vi "Run.vi"(8 "error in (no error)":errorcluster, 11 "Channel in":refnum<class "Channel.lvclass">) -> (0 "error out":errorcluster, 3 "Channel out":refnum<class "Channel.lvclass">)   [LabVIEW 2018, in "Channel.lvclass"]
doc: "Run the channel"
uses:
  Channel.lvclass
  Channel.lvclass/Channel.ctl
  Header content/Header content.lvclass/Header content.ctl
  Server/Server.lvclass/Server.ctl
  Simulated_CCD_Camera/Simulated Camera.lvclass/Simulated Camera.ctl
  Server/Server.lvclass
  RxTx/CCS_RxTx.lvclass
  State Machine/CCS_State Machine.lvclass
  Simulated_CCD_Camera/Simulated Camera.lvclass
  Header content/Header content.lvclass
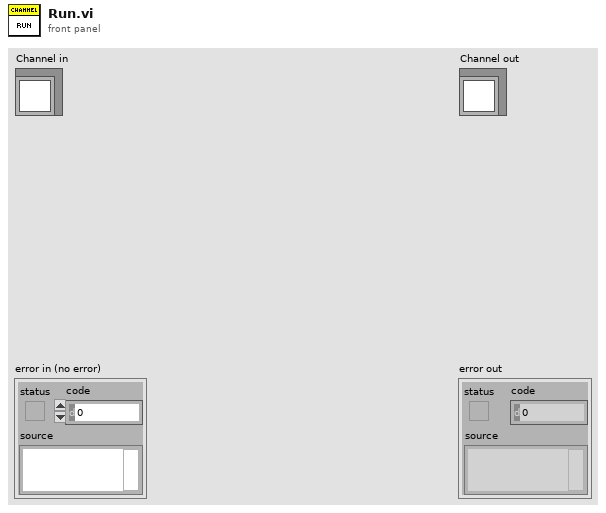
[diagram p1: front panel]
types:
  T1 = cluster{"PREAMP":u16, "READOUT_RATE":u16, "EM_GAIN":u16, "VERTICAL_SHIFT_SPEED":u16, "READ_MODE":u16, "FRAME_TRANSFER":bool, "VERTICAL_CLOCK_VOLTAGE":u16, "ACQUISITION_MODE":u16, "AD_CHANNEL":u16, "EM_MODE":u16, "SHUTTER_TTL":u16, "SHUTTER_OPENING_TIME":u16, "SHUTTER_CLOSING_TIME":u16, "SHUTTER_MODE":u16, "TRIGGER_MODE":u16, "VBIN":u16, "INITIAL_LINE":u16, "INITIAL_COLUMN":u16, "FINAL_LINE":u16, "FINAL_COLUMN":u16, "HBIN":u16}
  T2 = cluster{"CYCLES_DONE":u16, "LAST_IMAGE_NAME":string, "USED_DISK_SPACE":u16, "FRAMES_DONE":u16, "CCD_STATUS":string, "CURRENT_TEMPERATURE":i16, "TEMPERATURE_STATUS":string, "FRAME_EXPOSURE_TIME":sgl, "ERROR":bool, "SERIAL_NUMBER":u16, "ACQUIRING":bool, "IMAGE_INDEX":u32, "SEQS_DONE":u16}
  T3 = cluster{"COOLER_POWER_STATUS":u16, "TEMP":i32, "EXPTIME":dbl, "#FRAMES":u32, "#CYCLES":u32, "#SEQS":u32, "WAVEPLATE_POS":u16}
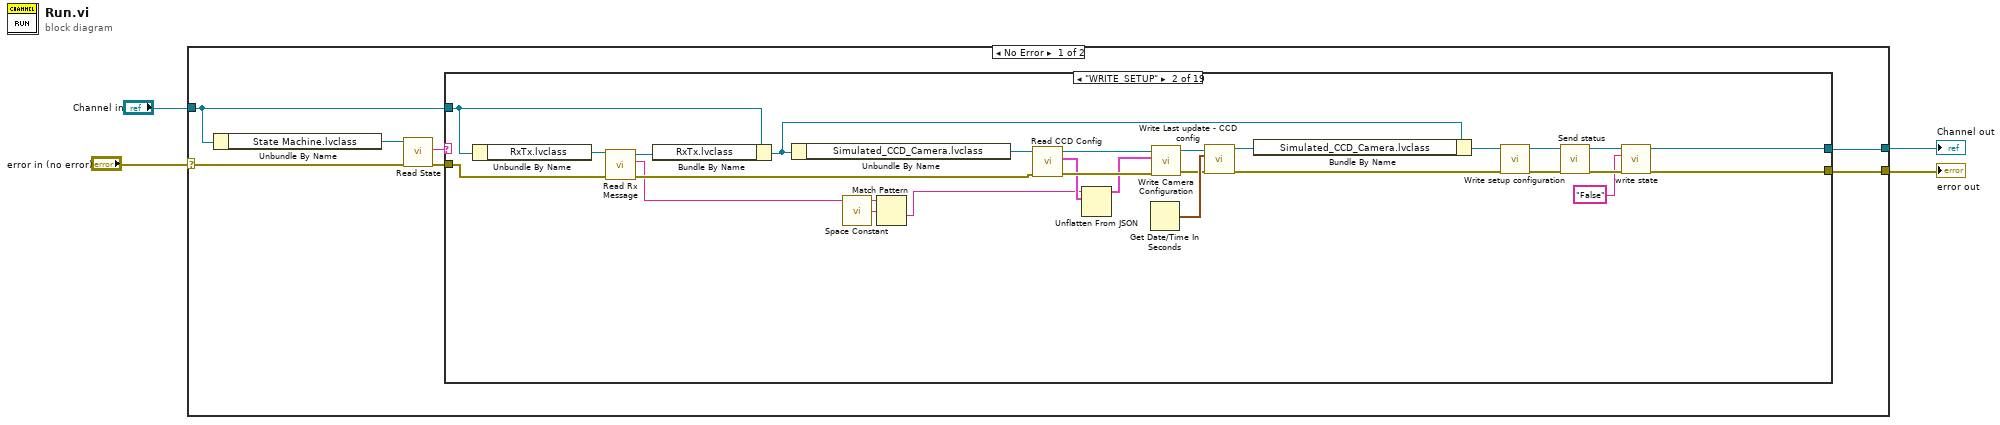
[diagram p0: block diagram]
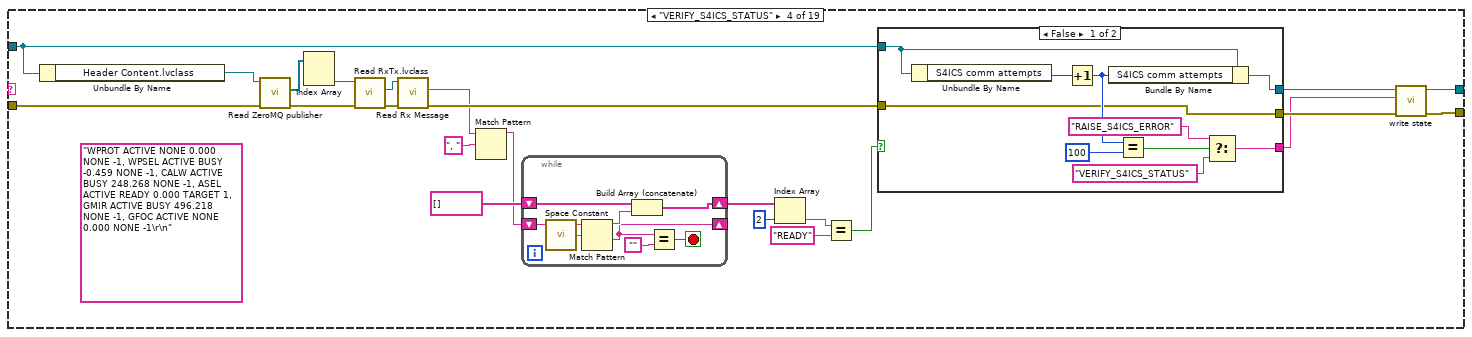
[diagram p4: hidden frame]
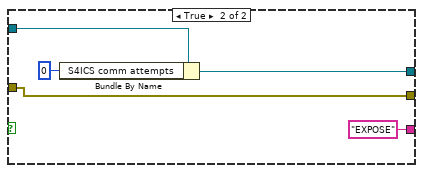
[diagram p5: hidden frame]
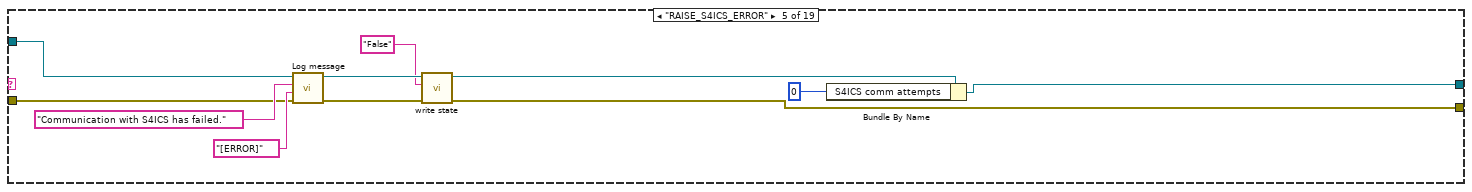
[diagram p6: hidden frame]
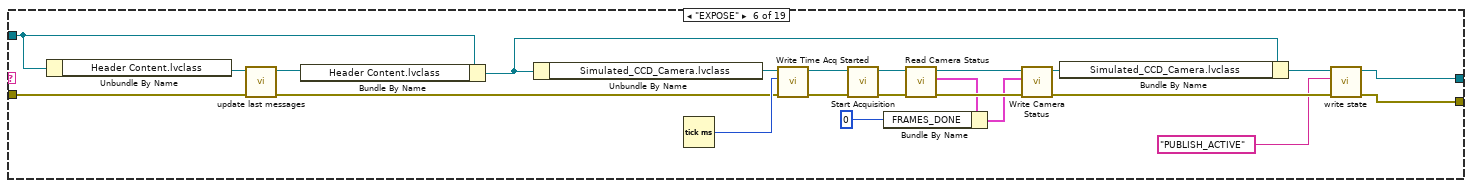
[diagram p7: hidden frame]
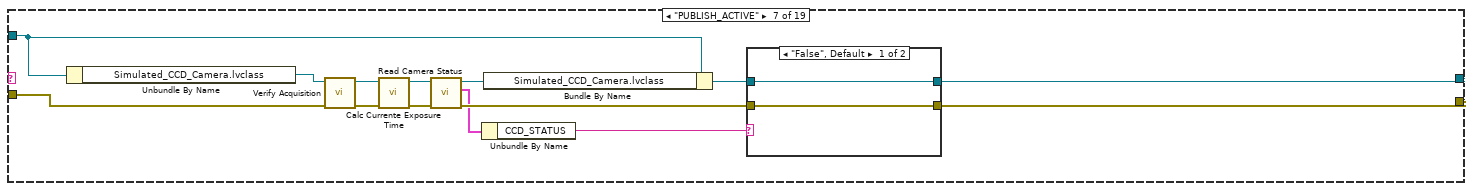
[diagram p8: hidden frame]
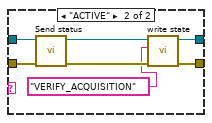
[diagram p9: hidden frame]
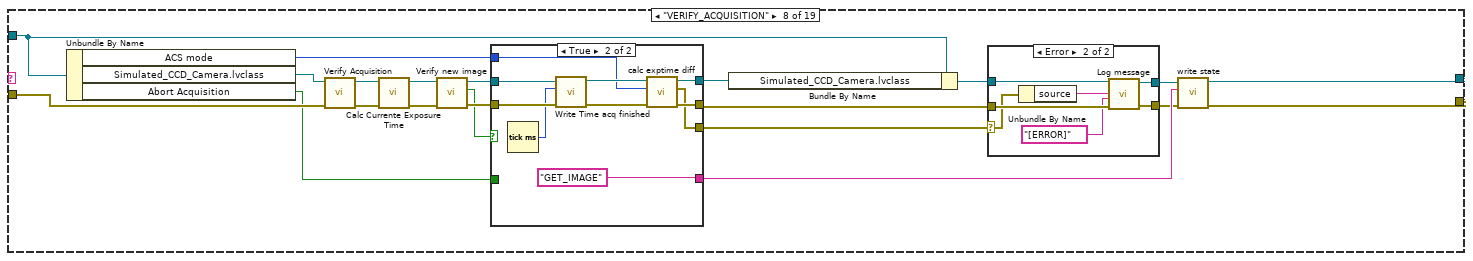
[diagram p10: hidden frame]
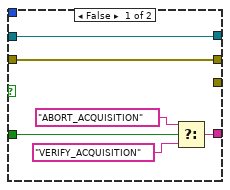
[diagram p12: hidden frame]
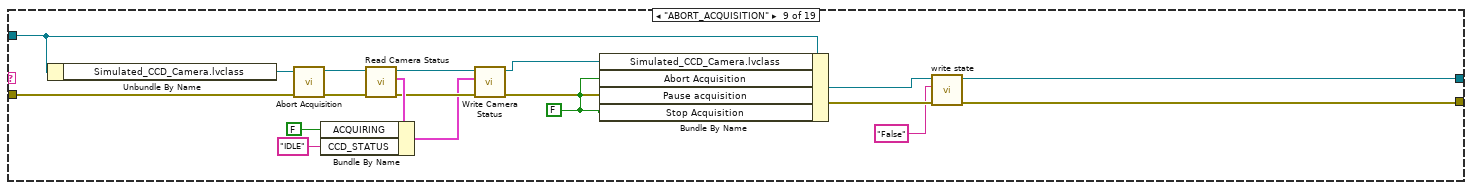
[diagram p13: hidden frame]
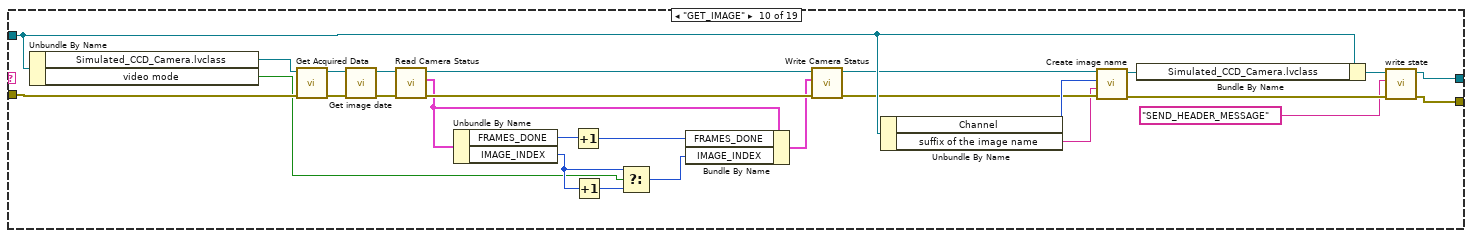
[diagram p14: hidden frame]
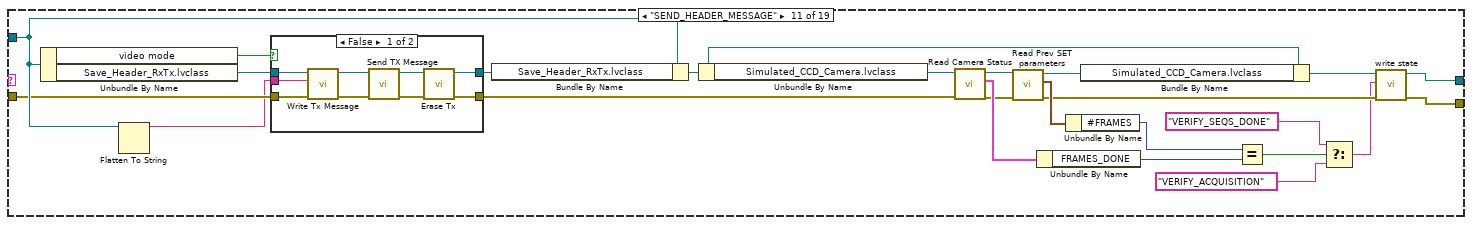
[diagram p15: hidden frame]
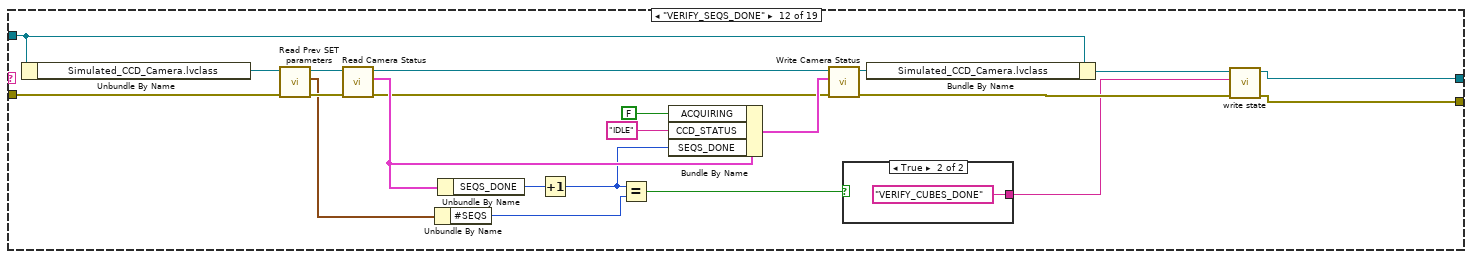
[diagram p17: hidden frame]
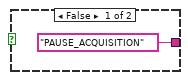
[diagram p18: hidden frame]
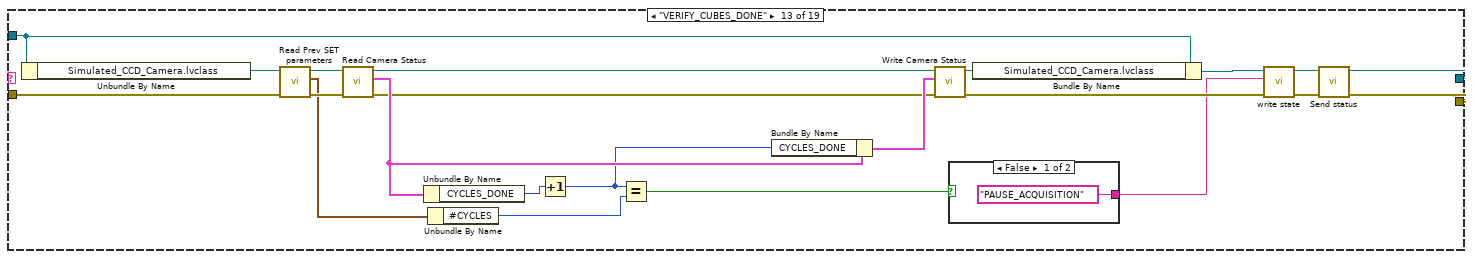
[diagram p19: hidden frame]
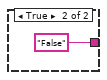
[diagram p20: hidden frame]
diagram:
  n1 = case shown="No Error" "error in (no error)" {
    selector: "error in (no error)" -> [w7 w489]
    tunnel: [w11 w489] -> w3
    tunnel: [w9 w488] -> w1
    tunnel: "Channel in" -> [w10 w488]
    frame No Error {
      n2 = Unbundle By Name(w10) -> ("State Machine.lvclass"=w8:refnum<class "CCS_State Machine.lvclass">)
      n3 = call-dynamic "Read State.vi"("error in (no error)"=w7, "State Machine in"=w8) -> ("error out"=w6:errorcluster, "State"=w5:string)  [unwired: 7 in, 1 out]
      n4 = case shown="\"WRITE_SETUP\"" w5 {
        tunnel: w6 -> [w12 w38 w41 w60 w96 w113 w133 w162 w200 w236 w246 w284 w309 w323 w329 w353 w365 w384 w401]
        tunnel: [w12 w23 w41 w46 w90 w104 w129 w158 w193 w210 w237 w272 w301 w322 w336 w352 w366 w384 w391] -> w11
        tunnel: [w13 w24 w42 w47 w91 w105 w130 w159 w194 w211 w238 w273 w302 w321 w337 w351 w367 w385 w392] -> w9
        tunnel: w10 -> [w13 w40 w42 w50 w97 w112 w136 w166 w199 w229 w248 w288 w315 w324 w349 w354 w364 w385 w403]
        frame "False", Default {
        }
        frame "WRITE_SETUP" {
          n5 = Unbundle By Name(w40) -> ("RxTx.lvclass"=w39:refnum<class "CCS_RxTx.lvclass">)
          n6 = call "Read Rx Message.vi"("error in (no error)"=w38, "RxTx in"=w39) -> ("error out"=w33:errorcluster, "Rx Message"=w15:string, "RxTx out"=w37:refnum<class "CCS_RxTx.lvclass">)  [unwired: 7 in]
          n7 = Bundle By Name(cluster=w40, "RxTx.lvclass"=w37) -> (w28:refnum<class "Channel.lvclass">)
          n8 = Unbundle By Name(w28) -> ("Simulated_CCD_Camera.lvclass"=w36:refnum<class "Simulated Camera.lvclass">)
          n9 = call <vilib>:"Space Constant.vi"() -> ("String"=w16:string)
          n10 = Match Pattern(string=w15, regular expression=w16) -> (after substring=w14:string)  [unwired: 1 in, 3 out]
          n11 = call "Read CCD Config.vi"("error in (no error)"=w33, "CCDCamera in"=w36) -> ("error out"=w34:errorcluster, "CCD Config"=w32:T1, "CCDCamera out"=w35:refnum<class "Simulated Camera.lvclass">)  [unwired: 7 in]
          n12 = Unflatten From JSON(JSON string=w14, type and defaults=w32) -> (value=w31:T1)  [unwired: 5 in, 1 out]
          n13 = Get Date/Time In Seconds() -> (seconds since 1Jan1904=w30:timestamp)
          n14 = call-dynamic "Write Camera Configuration.vi"("error in (no error)"=w34, "CCD Config"=w31, "CCDCamera in"=w35) -> ("error out"=w21:errorcluster, "CCDCamera out"=w22:refnum<class "Simulated Camera.lvclass">)  [unwired: 7 in]
          n15 = call-dynamic "Write Last update - CCD config.vi"("error in (no error)"=w21, "Last update - CCD config"=w30, "Simulated_CCD_Camera in"=w22) -> ("error out"=w19:errorcluster, "Simulated_CCD_Camera out"=w29:refnum<class "Simulated Camera.lvclass">)  [unwired: 7 in]
          n16 = Bundle By Name(cluster=w28, "Simulated_CCD_Camera.lvclass"=w29) -> (w20:refnum<class "Channel.lvclass">)
          n17 = call "Write setup configuration.vi"("error in (no error)"=w19, "Channel in"=w20) -> ("error out"=w18:errorcluster, "Channel out"=w17:refnum<class "Channel.lvclass">)  [unwired: 8 in]
          n18 = call "Send status.vi"("error in (no error)"=w18, "Channel in"=w17) -> ("error out"=w26:errorcluster, "Channel out"=w27:refnum<class "Channel.lvclass">)  [unwired: 8 in]
          n19 = call "write state.vi"("error in (no error)"=w26, "state"="False", "Channel in"=w27) -> ("error out"=w23:errorcluster, "Channel out"=w24:refnum<class "Channel.lvclass">)  [unwired: 7 in]
        }
        frame "---------------------------------" {
        }
        frame "VERIFY_S4ICS_STATUS" {
          (unwired) "WPROT ACTIVE NONE 0.000 NONE -1, WPSEL ACTIVE BUSY -0.459 NONE -1, CALW ACTIVE BUSY 248.268 NONE -1, ASEL ACTIVE READY 0.000 TARGET 1, GMIR ACTIVE BUSY 496.218 NONE -1, GFOC ACTIVE NONE 0.000 NONE -1\r\n" ("search string/char (-)")
          n20 = Unbundle By Name(w50) -> ("Header Content.lvclass"=w59:refnum<class "Header content.lvclass">)
          n21 = call "Read ZeroMQ publisher.vi"("error in (no error)"=w60, "Header content in"=w59) -> ("error out"=w62:errorcluster, "ZeroMQ publisher"=w65:refnum<class "Server.lvclass">[])  [unwired: 7 in, 1 out]
          n22 = Index Array(array=w65) -> (element #2=w61:refnum<class "Server.lvclass">)  [unwired: 2 in, 1 out]
          n23 = call "Read RxTx.lvclass.vi"("error in (no error)"=w62, "Server in"=w61) -> ("error out"=w63:errorcluster, "RxTx.lvclass"=w64:refnum<class "CCS_RxTx.lvclass">)  [unwired: 7 in, 1 out]
          n24 = call "Read Rx Message.vi"("error in (no error)"=w63, "RxTx in"=w64) -> ("error out"=w49:errorcluster, "Rx Message"=w43:string)  [unwired: 7 in, 1 out]
          n25 = Match Pattern(string=w43, regular expression=", " ("search string/char (-)")) -> (before substring=w56:string)  [unwired: 1 in, 3 out]
          n26 = while {
            shift-right: [w85] -> w52
            shift-left: string[] [] -> [w86]
            shift-right: [w82] -> _
            shift-left: w56 -> [w84]
            stop <- w87 stop-if-true
            n27 = call <vilib>:"Space Constant.vi"() -> ("String"=w81:string)
            n28 = Match Pattern(string=w84, regular expression=w81) -> (before substring=w83:string, after substring=w82:string)  [unwired: 1 in, 2 out]
            n29 = Build Array (concatenate)(w86, w83) -> (w85:string[])
            n30 = Equal?(x=w82, y="") -> (x = y?=w87:bool)
          }
          n31 = Index Array(array=w52, index=2) -> (element=w54:string)
          n32 = Equal?(x=w54, y="READY") -> (x = y?=w51:bool)
          n33 = case shown="False" w51 {
            tunnel: w50 -> [w75 w80]
            tunnel: w49 -> [w68 w79]
            tunnel: [w67 w78] -> w48
            tunnel: [w68 w79] -> w45
            tunnel: [w66 "EXPOSE" ("y")] -> w44
            frame False {
              n34 = Unbundle By Name(w75) -> ("S4ICS comm attempts"=w74:u8)
              n35 = Increment(x=w74) -> (x+1=w73:u8)
              n36 = Bundle By Name(cluster=w75, "S4ICS comm attempts"=w73) -> (w67:refnum<class "Channel.lvclass">)
              n37 = Equal?(x=w73, y=100) -> (x = y?=w71:bool)
              n38 = Select(t="RAISE_S4ICS_ERROR" ("y"), s=w71, f="VERIFY_S4ICS_STATUS" ("y")) -> (s? t:f=w66:string)
            }
            frame True {
              n39 = Bundle By Name(cluster=w80, "S4ICS comm attempts"=u8 0) -> (w78:refnum<class "Channel.lvclass">)
            }
          }
          n40 = call "write state.vi"("error in (no error)"=w45, "state"=w44, "Channel in"=w48) -> ("error out"=w46:errorcluster, "Channel out"=w47:refnum<class "Channel.lvclass">)  [unwired: 7 in]
        }
        frame "RAISE_S4ICS_ERROR" {
          n41 = call "Log message.vi"("error in (no error)"=w96, "message type"="[ERROR]", "String"="Communication with S4ICS has failed.", "Channel in"=w97) -> ("error out"=w93:errorcluster, "Channel out"=w94:refnum<class "Channel.lvclass">)  [unwired: 6 in]
          n42 = call "write state.vi"("error in (no error)"=w93, "state"="False", "Channel in"=w94) -> ("error out"=w90:errorcluster, "Channel out"=w92:refnum<class "Channel.lvclass">)  [unwired: 7 in]
          n43 = Bundle By Name(cluster=w92, "S4ICS comm attempts"=u8 0) -> (w91:refnum<class "Channel.lvclass">)
        }
        frame "EXPOSE" {
          n44 = Unbundle By Name(w112) -> ("Header Content.lvclass"=w114:refnum<class "Header content.lvclass">)
          n45 = call "update last messages.vi"("error in (no error)"=w113, "Header content in"=w114) -> ("error out"=w110:errorcluster, "Header content out"=w111:refnum<class "Header content.lvclass">)  [unwired: 8 in]
          n46 = Bundle By Name(cluster=w112, "Header Content.lvclass"=w111) -> (w109:refnum<class "Channel.lvclass">)
          n47 = Unbundle By Name(w109) -> ("Simulated_CCD_Camera.lvclass"=w122:refnum<class "Simulated Camera.lvclass">)
          n48 = Tick Count (ms)() -> (millisecond timer value=w121:u32)
          n49 = call "Write Time Acq Started.vi"("error in (no error)"=w110, "Time Acq Started"=w121, "Simulated_CCD_Camera in"=w122) -> ("error out"=w100:errorcluster, "Simulated_CCD_Camera out"=w103:refnum<class "Simulated Camera.lvclass">)  [unwired: 7 in]
          n50 = call-dynamic "Start Acquisition.vi"("error in (no error)"=w100, "CCDCamera in"=w103) -> ("error out"=w101:errorcluster, "CCDCamera out"=w102:refnum<class "Simulated Camera.lvclass">)  [unwired: 8 in]
          n51 = call "Read Camera Status.vi"("error in (no error)"=w101, "CCDCamera in"=w102) -> ("error out"=w119:errorcluster, "Camera Status"=w117:T2, "CCDCamera out"=w118:refnum<class "Simulated Camera.lvclass">)  [unwired: 7 in]
          n52 = Bundle By Name(cluster=w117, "FRAMES_DONE"=u16 0) -> (w116:T2)
          n53 = call "Write Camera Status.vi"("error in (no error)"=w119, "Camera Status"=w116, "CCDCamera in"=w118) -> ("error out"=w107:errorcluster, "CCDCamera out"=w120:refnum<class "Simulated Camera.lvclass">)  [unwired: 7 in]
          n54 = Bundle By Name(cluster=w109, "Simulated_CCD_Camera.lvclass"=w120) -> (w108:refnum<class "Channel.lvclass">)
          n55 = call "write state.vi"("error in (no error)"=w107, "state"="PUBLISH_ACTIVE", "Channel in"=w108) -> ("error out"=w104:errorcluster, "Channel out"=w105:refnum<class "Channel.lvclass">)  [unwired: 7 in]
        }
        frame "PUBLISH_ACTIVE" {
          n56 = Unbundle By Name(w136) -> ("Simulated_CCD_Camera.lvclass"=w134:refnum<class "Simulated Camera.lvclass">)
          n57 = call-dynamic "Verify Acquisition.vi"("error in (no error)"=w133, "CCDCamera in"=w134) -> ("error out"=w135:errorcluster, "CCDCamera out"=w132:refnum<class "Simulated Camera.lvclass">)  [unwired: 8 in]
          n58 = call-dynamic "Calc Currente Exposure Time.vi"("error in (no error)"=w135, "CCDCamera in"=w132) -> ("error out"=w128:errorcluster, "CCDCamera out"=w127:refnum<class "Simulated Camera.lvclass">)  [unwired: 8 in]
          n59 = call "Read Camera Status.vi"("error in (no error)"=w128, "CCDCamera in"=w127) -> ("error out"=w125:errorcluster, "Camera Status"=w124:T2, "CCDCamera out"=w126:refnum<class "Simulated Camera.lvclass">)  [unwired: 7 in]
          n60 = Unbundle By Name(w124) -> ("CCD_STATUS"=w123:string)
          n61 = Bundle By Name(cluster=w136, "Simulated_CCD_Camera.lvclass"=w126) -> (w131:refnum<class "Channel.lvclass">)
          n62 = case shown="\"False\", Default" w123 {
            tunnel: w131 -> [w138 w141]
            tunnel: [w138 w145] -> w130
            tunnel: [w137 w144] -> w129
            tunnel: w125 -> [w137 w140]
            frame "False", Default {
            }
            frame "ACTIVE" {
              n63 = call "Send status.vi"("error in (no error)"=w140, "Channel in"=w141) -> ("error out"=w143:errorcluster, "Channel out"=w142:refnum<class "Channel.lvclass">)  [unwired: 8 in]
              n64 = call "write state.vi"("error in (no error)"=w143, "state"="VERIFY_ACQUISITION", "Channel in"=w142) -> ("error out"=w144:errorcluster, "Channel out"=w145:refnum<class "Channel.lvclass">)  [unwired: 7 in]
            }
          }
        }
        frame "VERIFY_ACQUISITION" {
          n65 = Unbundle By Name(w166) -> ("ACS mode"=w151:u16, "Simulated_CCD_Camera.lvclass"=w163:refnum<class "Simulated Camera.lvclass">, "Abort Acquisition"=w154:bool)
          n66 = call-dynamic "Verify Acquisition.vi"("error in (no error)"=w162, "CCDCamera in"=w163) -> ("error out"=w164:errorcluster, "CCDCamera out"=w161:refnum<class "Simulated Camera.lvclass">)  [unwired: 8 in]
          n67 = call-dynamic "Calc Currente Exposure Time.vi"("error in (no error)"=w164, "CCDCamera in"=w161) -> ("error out"=w165:errorcluster, "CCDCamera out"=w160:refnum<class "Simulated Camera.lvclass">)  [unwired: 8 in]
          n68 = call-dynamic "Verify new image.vi"("error in (no error)"=w165, "CCDCamera in"=w160) -> ("error out"=w156:errorcluster, "New Images ?"=w153:bool, "CCDCamera out"=w157:refnum<class "Simulated Camera.lvclass">)  [unwired: 7 in]
          n69 = case shown="True" w153 {
            tunnel: w157 -> [w181 w191]
            tunnel: w156 -> [w180 w190]
            tunnel: [w181 w185] -> w155
            tunnel: [w180 w186] -> w147
            tunnel: w154 -> [w177 _]
            tunnel: [w176 "GET_IMAGE"] -> w152
            tunnel: w151 -> [_ w183]
            tunnel: [_ w182] -> w146
            frame False {
              n70 = Select(t="ABORT_ACQUISITION", s=w177, f="VERIFY_ACQUISITION") -> (s? t:f=w176:string)
            }
            frame True {
              n71 = Tick Count (ms)() -> (millisecond timer value=w188:u32)
              n72 = call "Write Time acq finished.vi"("error in (no error)"=w190, "Time acq finished"=w188, "Simulated_CCD_Camera in"=w191) -> ("error out"=w187:errorcluster, "Simulated_CCD_Camera out"=w184:refnum<class "Simulated Camera.lvclass">)  [unwired: 7 in]
              n73 = call "calc exptime diff.vi"("error in (no error)"=w187, "ACS mode"=w183, "Simulated_CCD_Camera in"=w184) -> (0:"error out"=w186:errorcluster, 2:"error out"=w182:errorcluster, "Simulated_CCD_Camera out"=w185:refnum<class "Simulated Camera.lvclass">)  [unwired: 6 in]
            }
          }
          n74 = Bundle By Name(cluster=w166, "Simulated_CCD_Camera.lvclass"=w155) -> (w150:refnum<class "Channel.lvclass">)
          n75 = case shown="Error" w146 {
            selector: w146 -> [_ w170]
            tunnel: w150 -> [w168 w175]
            tunnel: [w168 w174] -> w149
            tunnel: [w167 w173] -> w148
            tunnel: w147 -> [w167 w172]
            frame No Error {
            }
            frame Error {
              n76 = Unbundle By Name(w170) -> ("source"=w169:string)
              n77 = call "Log message.vi"("error in (no error)"=w172, "message type"="[ERROR]", "String"=w169, "Channel in"=w175) -> ("error out"=w173:errorcluster, "Channel out"=w174:refnum<class "Channel.lvclass">)  [unwired: 6 in]
            }
          }
          n78 = call "write state.vi"("error in (no error)"=w148, "state"=w152, "Channel in"=w149) -> ("error out"=w158:errorcluster, "Channel out"=w159:refnum<class "Channel.lvclass">)  [unwired: 7 in]
        }
        frame "ABORT_ACQUISITION" {
          w192 = FALSE ("Acquiring")
          n79 = Unbundle By Name(w199) -> ("Simulated_CCD_Camera.lvclass"=w201:refnum<class "Simulated Camera.lvclass">)
          n80 = call-dynamic "Abort Acquisition.vi"("error in (no error)"=w200, "CCDCamera in"=w201) -> ("error out"=w206:errorcluster, "CCDCamera out"=w207:refnum<class "Simulated Camera.lvclass">)  [unwired: 8 in]
          n81 = call "Read Camera Status.vi"("error in (no error)"=w206, "CCDCamera in"=w207) -> ("error out"=w204:errorcluster, "Camera Status"=w209:T2, "CCDCamera out"=w205:refnum<class "Simulated Camera.lvclass">)  [unwired: 7 in]
          n82 = Bundle By Name(cluster=w209, "ACQUIRING"=FALSE ("Acquiring"), "CCD_STATUS"="IDLE" ("STATUS")) -> (w203:T2)
          n83 = call "Write Camera Status.vi"("error in (no error)"=w204, "Camera Status"=w203, "CCDCamera in"=w205) -> ("error out"=w196:errorcluster, "CCDCamera out"=w198:refnum<class "Simulated Camera.lvclass">)  [unwired: 7 in]
          n84 = Bundle By Name(cluster=w199, "Simulated_CCD_Camera.lvclass"=w198, "Abort Acquisition"=w192, "Pause acquisition"=w192, "Stop Acquisition"=w192) -> (w197:refnum<class "Channel.lvclass">)
          n85 = call "write state.vi"("error in (no error)"=w196, "state"="False", "Channel in"=w197) -> ("error out"=w193:errorcluster, "Channel out"=w194:refnum<class "Channel.lvclass">)  [unwired: 7 in]
        }
        frame "GET_IMAGE" {
          n86 = Unbundle By Name(w229) -> ("Simulated_CCD_Camera.lvclass"=w218:refnum<class "Simulated Camera.lvclass">, "video mode"=w215:bool)
          n87 = call-dynamic "Get Acquired Data.vi"("error in (no error)"=w236, "CCDCamera in"=w218) -> ("error out"=w221:errorcluster, "CCDCamera out"=w224:refnum<class "Simulated Camera.lvclass">)  [unwired: 8 in]
          n88 = call-dynamic "Get image date.vi"("error in (no error)"=w221, "Simulated_CCD_Camera in"=w224) -> ("error out"=w222:errorcluster, "Simulated_CCD_Camera out"=w223:refnum<class "Simulated Camera.lvclass">)  [unwired: 8 in]
          n89 = call "Read Camera Status.vi"("error in (no error)"=w222, "CCDCamera in"=w223) -> ("error out"=w235:errorcluster, "Camera Status"=w231:T2, "CCDCamera out"=w234:refnum<class "Simulated Camera.lvclass">)  [unwired: 7 in]
          n90 = Unbundle By Name(w231) -> ("FRAMES_DONE"=w233:u16, "IMAGE_INDEX"=w216:u32)
          n91 = Increment(x=w233) -> (x+1=w219:u16)
          n92 = Increment(x=w216) -> (x+1=w217:u32)
          n93 = Select(t=w216, s=w215, f=w217) -> (s? t:f=w220:u32)
          n94 = Bundle By Name(cluster=w231, "FRAMES_DONE"=w219, "IMAGE_INDEX"=w220) -> (w232:T2)
          n95 = call "Write Camera Status.vi"("error in (no error)"=w235, "Camera Status"=w232, "CCDCamera in"=w234) -> ("error out"=w226:errorcluster, "CCDCamera out"=w227:refnum<class "Simulated Camera.lvclass">)  [unwired: 7 in]
          n96 = Unbundle By Name(w229) -> ("Channel"=w228:u8, "suffix of the image name"=w225:string)
          n97 = call "Create image name.vi"("error in (no error)"=w226, "Suffix"=w225, "Channel"=w228, "Simulated_CCD_Camera in"=w227) -> ("error out"=w213:errorcluster, "Simulated_CCD_Camera out"=w230:refnum<class "Simulated Camera.lvclass">)  [unwired: 6 in]
          n98 = Bundle By Name(cluster=w229, "Simulated_CCD_Camera.lvclass"=w230) -> (w214:refnum<class "Channel.lvclass">)
          n99 = call "write state.vi"("error in (no error)"=w213, "state"="SEND_HEADER_MESSAGE", "Channel in"=w214) -> ("error out"=w210:errorcluster, "Channel out"=w211:refnum<class "Channel.lvclass">)  [unwired: 7 in]
        }
        frame "SEND_HEADER_MESSAGE" {
          n100 = Unbundle By Name(w248) -> ("video mode"=w242:bool, "Save_Header_RxTx.lvclass"=w247:refnum<class "CCS_RxTx.lvclass">)
          n101 = Flatten To String(anything=w248) -> (data string=w243:string)  [unwired: 3 in, 2 out]
          n102 = case shown="False" w242 {
            tunnel: w247 -> [w269 w271]
            tunnel: w246 -> [w266 w270]
            tunnel: [w264 w271] -> w245
            tunnel: [w262 w270] -> w244
            tunnel: w243 -> [w261 _]
            frame False {
              n103 = call "Write Tx Message.vi"("error in (no error)"=w266, "Tx Message"=w261, "RxTx in"=w269) -> ("error out"=w267:errorcluster, "RxTx out"=w268:refnum<class "CCS_RxTx.lvclass">)  [unwired: 7 in]
              n104 = call "Send TX Message.vi"("error in (no error)"=w267, "RxTx in"=w268) -> ("error out"=w263:errorcluster, "RxTx out"=w265:refnum<class "CCS_RxTx.lvclass">)  [unwired: 8 in]
              n105 = call "Erase Tx.vi"("error in (no error)"=w263, "RxTx in"=w265) -> ("error out"=w262:errorcluster, "RxTx out"=w264:refnum<class "CCS_RxTx.lvclass">)  [unwired: 8 in]
            }
            frame True {
            }
          }
          n106 = Bundle By Name(cluster=w248, "Save_Header_RxTx.lvclass"=w245) -> (w258:refnum<class "Channel.lvclass">)
          n107 = Unbundle By Name(w258) -> ("Simulated_CCD_Camera.lvclass"=w255:refnum<class "Simulated Camera.lvclass">)
          n108 = call "Read Camera Status.vi"("error in (no error)"=w244, "CCDCamera in"=w255) -> ("error out"=w251:errorcluster, "Camera Status"=w254:T2, "CCDCamera out"=w253:refnum<class "Simulated Camera.lvclass">)  [unwired: 7 in]
          n109 = call-dynamic "Read Prev SET parameters.vi"("error in (no error)"=w251, "Simulated_CCD_Camera in"=w253) -> ("error out"=w240:errorcluster, "Prev SET parameters"=w250:T3, "Simulated_CCD_Camera out"=w252:refnum<class "Simulated Camera.lvclass">)  [unwired: 7 in]
          n110 = Unbundle By Name(w254) -> ("FRAMES_DONE"=w260:u16)
          n111 = Unbundle By Name(w250) -> ("#FRAMES"=w249:u32)
          n112 = Bundle By Name(cluster=w258, "Simulated_CCD_Camera.lvclass"=w252) -> (w241:refnum<class "Channel.lvclass">)
          n113 = Equal?(x=w249, y=w260) -> (x = y?=w259:bool)
          n114 = Select(t="VERIFY_SEQS_DONE", s=w259, f="VERIFY_ACQUISITION") -> (s? t:f=w239:string)
          n115 = call "write state.vi"("error in (no error)"=w240, "state"=w239, "Channel in"=w241) -> ("error out"=w237:errorcluster, "Channel out"=w238:refnum<class "Channel.lvclass">)  [unwired: 7 in]
        }
        frame "VERIFY_SEQS_DONE" {
          n116 = Unbundle By Name(w288) -> ("Simulated_CCD_Camera.lvclass"=w287:refnum<class "Simulated Camera.lvclass">)
          n117 = call-dynamic "Read Prev SET parameters.vi"("error in (no error)"=w284, "Simulated_CCD_Camera in"=w287) -> ("error out"=w285:errorcluster, "Prev SET parameters"=w283:T3, "Simulated_CCD_Camera out"=w286:refnum<class "Simulated Camera.lvclass">)  [unwired: 7 in]
          n118 = call "Read Camera Status.vi"("error in (no error)"=w285, "CCDCamera in"=w286) -> ("error out"=w279:errorcluster, "Camera Status"=w293:T2, "CCDCamera out"=w280:refnum<class "Simulated Camera.lvclass">)  [unwired: 7 in]
          n119 = Unbundle By Name(w283) -> ("#SEQS"=w282:u32)
          n120 = Unbundle By Name(w293) -> ("SEQS_DONE"=w292:u16)
          n121 = Increment(x=w292) -> (x+1=w290:u16)
          n122 = Equal?(x=w290, y=w282) -> (x = y?=w289:bool)
          n123 = Bundle By Name(cluster=w293, "ACQUIRING"=FALSE, "CCD_STATUS"="IDLE", "SEQS_DONE"=w290) -> (w291:T2)
          n124 = call "Write Camera Status.vi"("error in (no error)"=w279, "Camera Status"=w291, "CCDCamera in"=w280) -> ("error out"=w275:errorcluster, "CCDCamera out"=w281:refnum<class "Simulated Camera.lvclass">)  [unwired: 7 in]
          n125 = case shown="True" w289 {
            tunnel: ["PAUSE_ACQUISITION" "VERIFY_CUBES_DONE"] -> w274
            frame False {
            }
            frame True {
            }
          }
          n126 = Bundle By Name(cluster=w288, "Simulated_CCD_Camera.lvclass"=w281) -> (w276:refnum<class "Channel.lvclass">)
          n127 = call "write state.vi"("error in (no error)"=w275, "state"=w274, "Channel in"=w276) -> ("error out"=w272:errorcluster, "Channel out"=w273:refnum<class "Channel.lvclass">)  [unwired: 7 in]
        }
        frame "VERIFY_CUBES_DONE" {
          n128 = Unbundle By Name(w315) -> ("Simulated_CCD_Camera.lvclass"=w312:refnum<class "Simulated Camera.lvclass">)
          n129 = call-dynamic "Read Prev SET parameters.vi"("error in (no error)"=w309, "Simulated_CCD_Camera in"=w312) -> ("error out"=w310:errorcluster, "Prev SET parameters"=w308:T3, "Simulated_CCD_Camera out"=w311:refnum<class "Simulated Camera.lvclass">)  [unwired: 7 in]
          n130 = call "Read Camera Status.vi"("error in (no error)"=w310, "CCDCamera in"=w311) -> ("error out"=w313:errorcluster, "Camera Status"=w317:T2, "CCDCamera out"=w314:refnum<class "Simulated Camera.lvclass">)  [unwired: 7 in]
          n131 = Unbundle By Name(w317) -> ("CYCLES_DONE"=w303:u16)
          n132 = Unbundle By Name(w308) -> ("#CYCLES"=w307:u32)
          n133 = Increment(x=w303) -> (x+1=w305:u16)
          n134 = Equal?(x=w305, y=w307) -> (x = y?=w304:bool)
          n135 = Bundle By Name(cluster=w317, "CYCLES_DONE"=w305) -> (w316:T2)
          n136 = call "Write Camera Status.vi"("error in (no error)"=w313, "Camera Status"=w316, "CCDCamera in"=w314) -> ("error out"=w297:errorcluster, "CCDCamera out"=w306:refnum<class "Simulated Camera.lvclass">)  [unwired: 7 in]
          n137 = case shown="False" w304 {
            tunnel: ["PAUSE_ACQUISITION" "False"] -> w296
            frame False {
            }
            frame True {
            }
          }
          n138 = Bundle By Name(cluster=w315, "Simulated_CCD_Camera.lvclass"=w306) -> (w300:refnum<class "Channel.lvclass">)
          n139 = call "write state.vi"("error in (no error)"=w297, "state"=w296, "Channel in"=w300) -> ("error out"=w298:errorcluster, "Channel out"=w299:refnum<class "Channel.lvclass">)  [unwired: 7 in]
          n140 = call "Send status.vi"("error in (no error)"=w298, "Channel in"=w299) -> ("error out"=w301:errorcluster, "Channel out"=w302:refnum<class "Channel.lvclass">)  [unwired: 8 in]
        }
        frame "PAUSE_ACQUISITION" {
          n141 = Unbundle By Name(w324) -> ("Pause acquisition"=w327:bool)
          n142 = Select(t="PAUSE_ACQUISITION", s=w327, f="STOP_ACQUISITION") -> (s? t:f=w320:string)
          n143 = call "write state.vi"("error in (no error)"=w323, "state"=w320, "Channel in"=w324) -> ("error out"=w322:errorcluster, "Channel out"=w321:refnum<class "Channel.lvclass">)  [unwired: 7 in]
        }
        frame "STOP_ACQUISITION" {
          n144 = Unbundle By Name(w349) -> ("Stop Acquisition"=w333:bool)
          n145 = Bundle By Name(cluster=w349, "Stop Acquisition"=FALSE) -> (w332:refnum<class "Channel.lvclass">)
          n146 = Select(t="False", s=w333, f="WAIT_EXPOSE_COMMAND") -> (s? t:f=w328:string)
          n147 = call "write state.vi"("error in (no error)"=w329, "state"=w328, "Channel in"=w332) -> ("error out"=w330:errorcluster, "Channel out"=w331:refnum<class "Channel.lvclass">)  [unwired: 7 in]
          n148 = Unbundle By Name(w331) -> ("Simulated_CCD_Camera.lvclass"=w345:refnum<class "Simulated Camera.lvclass">)
          n149 = Not(x=w333) -> (.not. x?=w334:bool)
          n150 = Select(t="WAITING_EXPOSE_COMMAND" ("CCD_STATUS"), s=w334, f="IDLE" ("CCD_STATUS")) -> (s? t:f=w339:string)
          n151 = call "Read Camera Status.vi"("error in (no error)"=w330, "CCDCamera in"=w345) -> ("error out"=w342:errorcluster, "Camera Status"=w344:T2, "CCDCamera out"=w341:refnum<class "Simulated Camera.lvclass">)  [unwired: 7 in]
          n152 = Bundle By Name(cluster=w344, "CCD_STATUS"=w339) -> (w343:T2)
          n153 = call "Write Camera Status.vi"("error in (no error)"=w342, "Camera Status"=w343, "CCDCamera in"=w341) -> ("error out"=w336:errorcluster, "CCDCamera out"=w340:refnum<class "Simulated Camera.lvclass">)  [unwired: 7 in]
          n154 = Bundle By Name(cluster=w331, "Simulated_CCD_Camera.lvclass"=w340) -> (w337:refnum<class "Channel.lvclass">)
        }
        frame "WAIT_EXPOSE_COMMAND" {
          n155 = Unbundle By Name(w354) -> ("wait expose command"=w355:bool)
          n156 = Select(t="STOP_ACQUISITION", s=w355, f="RESET_#SEQS") -> (s? t:f=w350:string)
          n157 = call "write state.vi"("error in (no error)"=w353, "state"=w350, "Channel in"=w354) -> ("error out"=w352:errorcluster, "Channel out"=w351:refnum<class "Channel.lvclass">)  [unwired: 7 in]
        }
        frame "RESET_#SEQS" {
          n158 = call "choose firs acquisition state.vi"("error in (no error)"=w365, "Channel in"=w364) -> ("error out"=w362:errorcluster, "verify S4ICS status"=w358:bool, "Channel out"=w363:refnum<class "Channel.lvclass">)  [unwired: 7 in]
          n159 = Select(t="VERIFY_S4ICS_STATUS", s=w358, f="EXPOSE") -> (s? t:f=w360:string)
          n160 = call "write state.vi"("error in (no error)"=w362, "state"=w360, "Channel in"=w363) -> ("error out"=w368:errorcluster, "Channel out"=w369:refnum<class "Channel.lvclass">)  [unwired: 7 in]
          n161 = Unbundle By Name(w369) -> ("Simulated_CCD_Camera.lvclass"=w380:refnum<class "Simulated Camera.lvclass">)
          n162 = call "Read Camera Status.vi"("error in (no error)"=w368, "CCDCamera in"=w380) -> ("error out"=w373:errorcluster, "Camera Status"=w381:T2, "CCDCamera out"=w372:refnum<class "Simulated Camera.lvclass">)  [unwired: 7 in]
          n163 = call-dynamic "Read Prev SET parameters.vi"("error in (no error)"=w373, "Simulated_CCD_Camera in"=w372) -> ("error out"=w370:errorcluster, "Prev SET parameters"=w379:T3, "Simulated_CCD_Camera out"=w371:refnum<class "Simulated Camera.lvclass">)  [unwired: 7 in]
          n164 = Unbundle By Name(w381) -> ("SEQS_DONE"=w375:u16)
          n165 = Unbundle By Name(w379) -> ("#SEQS"=w378:u32)
          n166 = Equal?(x=w375, y=w378) -> (x = y?=w377:bool)
          n167 = Select(t=0, s=w377, f=w375) -> (s? t:f=w374:i32)
          n168 = Bundle By Name(cluster=w381, "SEQS_DONE"=w374) -> (w383:T2)
          n169 = call "Write Camera Status.vi"("error in (no error)"=w370, "Camera Status"=w383, "CCDCamera in"=w371) -> ("error out"=w366:errorcluster, "CCDCamera out"=w382:refnum<class "Simulated Camera.lvclass">)  [unwired: 7 in]
          n170 = Bundle By Name(cluster=w369, "Simulated_CCD_Camera.lvclass"=w382) -> (w367:refnum<class "Channel.lvclass">)
        }
        frame "------------------------------" {
        }
        frame "SET" {
          n171 = Unbundle By Name(w403) -> ("RxTx.lvclass"=w400:refnum<class "CCS_RxTx.lvclass">)
          n172 = call "Read Rx Message.vi"("error in (no error)"=w401, "RxTx in"=w400) -> ("error out"=w402:errorcluster, "Rx Message"=w398:string)  [unwired: 7 in, 1 out]
          n173 = call <vilib>:"Space Constant.vi"() -> ("String"=w397:string)
          n174 = Match Pattern(string=w398, regular expression=w397) -> (after substring=w399:string)  [unwired: 1 in, 3 out]
          n175 = Match Pattern(string=w399, regular expression=w397) -> (before substring=w396:string, after substring=w395:string)  [unwired: 1 in, 2 out]
          n176 = case shown="\"SUFFIX\"" w396 {
            tunnel: [w405 w417 w430 w443 w455 w468 w481 w486] -> w387
            tunnel: w403 -> [w405 w418 w431 w444 w456 w469 w482 w487]
            tunnel: [w404 w410 w423 w436 w445 w461 w474 w485] -> w386
            tunnel: w402 -> [w404 w412 w425 w438 w453 w463 w476 w485]
            tunnel: w395 -> [_ w414 w427 w440 w447 w465 w478 w483]
            frame "False", Default {
            }
            frame "EXPTIME" {
              n177 = Unbundle By Name(w418) -> ("Simulated_CCD_Camera.lvclass"=w413:refnum<class "Simulated Camera.lvclass">)
              n178 = Fract/Exp String To Number(string=w414, default (0 dbl)=0.0) -> (number=w415:dbl)  [unwired: 2 in, 1 out]
              n179 = call-dynamic "Read SET parameters.vi"("error in (no error)"=w412, "Simulated_CCD_Camera in"=w413) -> ("error out"=w406:errorcluster, "New SET parameters"=w409:T3, "Simulated_CCD_Camera out"=w407:refnum<class "Simulated Camera.lvclass">)  [unwired: 7 in]
              n180 = Bundle By Name(cluster=w409, "EXPTIME"=w415) -> (w408:T3)
              n181 = call-dynamic "Write SET parameters.vi"("error in (no error)"=w406, "New SET parameters"=w408, "Simulated_CCD_Camera in"=w407) -> ("error out"=w410:errorcluster, "Simulated_CCD_Camera out"=w411:refnum<class "Simulated Camera.lvclass">)  [unwired: 7 in]
              n182 = Bundle By Name(cluster=w418, "Simulated_CCD_Camera.lvclass"=w411) -> (w417:refnum<class "Channel.lvclass">)
            }
            frame "#FRAMES" {
              n183 = Unbundle By Name(w431) -> ("Simulated_CCD_Camera.lvclass"=w426:refnum<class "Simulated Camera.lvclass">)
              n184 = Fract/Exp String To Number(string=w427, default (0 dbl)=u32 0) -> (number=w428:u32)  [unwired: 2 in, 1 out]
              n185 = call-dynamic "Read SET parameters.vi"("error in (no error)"=w425, "Simulated_CCD_Camera in"=w426) -> ("error out"=w419:errorcluster, "New SET parameters"=w422:T3, "Simulated_CCD_Camera out"=w420:refnum<class "Simulated Camera.lvclass">)  [unwired: 7 in]
              n186 = Bundle By Name(cluster=w422, "#FRAMES"=w428) -> (w421:T3)
              n187 = call-dynamic "Write SET parameters.vi"("error in (no error)"=w419, "New SET parameters"=w421, "Simulated_CCD_Camera in"=w420) -> ("error out"=w423:errorcluster, "Simulated_CCD_Camera out"=w424:refnum<class "Simulated Camera.lvclass">)  [unwired: 7 in]
              n188 = Bundle By Name(cluster=w431, "Simulated_CCD_Camera.lvclass"=w424) -> (w430:refnum<class "Channel.lvclass">)
            }
            frame "#CYCLES" {
              n189 = Unbundle By Name(w444) -> ("Simulated_CCD_Camera.lvclass"=w439:refnum<class "Simulated Camera.lvclass">)
              n190 = Fract/Exp String To Number(string=w440, default (0 dbl)=u32 0) -> (number=w441:u32)  [unwired: 2 in, 1 out]
              n191 = call-dynamic "Read SET parameters.vi"("error in (no error)"=w438, "Simulated_CCD_Camera in"=w439) -> ("error out"=w432:errorcluster, "New SET parameters"=w435:T3, "Simulated_CCD_Camera out"=w433:refnum<class "Simulated Camera.lvclass">)  [unwired: 7 in]
              n192 = Bundle By Name(cluster=w435, "#CYCLES"=w441) -> (w434:T3)
              n193 = call-dynamic "Write SET parameters.vi"("error in (no error)"=w432, "New SET parameters"=w434, "Simulated_CCD_Camera in"=w433) -> ("error out"=w436:errorcluster, "Simulated_CCD_Camera out"=w437:refnum<class "Simulated Camera.lvclass">)  [unwired: 7 in]
              n194 = Bundle By Name(cluster=w444, "Simulated_CCD_Camera.lvclass"=w437) -> (w443:refnum<class "Channel.lvclass">)
            }
            frame "WAVEPLATE_POS" {
              n195 = Unbundle By Name(w456) -> ("Simulated_CCD_Camera.lvclass"=w454:refnum<class "Simulated Camera.lvclass">)
              n196 = Decimal String To Number(string=w447) -> (number=w448:i32)  [unwired: 2 in, 1 out]
              n197 = call-dynamic "Read SET parameters.vi"("error in (no error)"=w453, "Simulated_CCD_Camera in"=w454) -> ("error out"=w449:errorcluster, "New SET parameters"=w452:T3, "Simulated_CCD_Camera out"=w450:refnum<class "Simulated Camera.lvclass">)  [unwired: 7 in]
              n198 = Bundle By Name(cluster=w452, "WAVEPLATE_POS"=w448) -> (w451:T3)
              n199 = call-dynamic "Write SET parameters.vi"("error in (no error)"=w449, "New SET parameters"=w451, "Simulated_CCD_Camera in"=w450) -> ("error out"=w445:errorcluster, "Simulated_CCD_Camera out"=w446:refnum<class "Simulated Camera.lvclass">)  [unwired: 7 in]
              n200 = Bundle By Name(cluster=w456, "Simulated_CCD_Camera.lvclass"=w446) -> (w455:refnum<class "Channel.lvclass">)
            }
            frame "TEMP" {
              n201 = Unbundle By Name(w469) -> ("Simulated_CCD_Camera.lvclass"=w464:refnum<class "Simulated Camera.lvclass">)
              n202 = Fract/Exp String To Number(string=w465, default (0 dbl)=0) -> (number=w466:i32)  [unwired: 2 in, 1 out]
              n203 = call-dynamic "Read SET parameters.vi"("error in (no error)"=w463, "Simulated_CCD_Camera in"=w464) -> ("error out"=w457:errorcluster, "New SET parameters"=w460:T3, "Simulated_CCD_Camera out"=w458:refnum<class "Simulated Camera.lvclass">)  [unwired: 7 in]
              n204 = Bundle By Name(cluster=w460, "TEMP"=w466) -> (w459:T3)
              n205 = call-dynamic "Write SET parameters.vi"("error in (no error)"=w457, "New SET parameters"=w459, "Simulated_CCD_Camera in"=w458) -> ("error out"=w461:errorcluster, "Simulated_CCD_Camera out"=w462:refnum<class "Simulated Camera.lvclass">)  [unwired: 7 in]
              n206 = Bundle By Name(cluster=w469, "Simulated_CCD_Camera.lvclass"=w462) -> (w468:refnum<class "Channel.lvclass">)
            }
            frame "COOLER_POWER_STATUS" {
              n207 = Unbundle By Name(w482) -> ("Simulated_CCD_Camera.lvclass"=w477:refnum<class "Simulated Camera.lvclass">)
              n208 = Fract/Exp String To Number(string=w478, default (0 dbl)=u16 0) -> (number=w479:u16)  [unwired: 2 in, 1 out]
              n209 = call-dynamic "Read SET parameters.vi"("error in (no error)"=w476, "Simulated_CCD_Camera in"=w477) -> ("error out"=w470:errorcluster, "New SET parameters"=w473:T3, "Simulated_CCD_Camera out"=w471:refnum<class "Simulated Camera.lvclass">)  [unwired: 7 in]
              n210 = Bundle By Name(cluster=w473, "COOLER_POWER_STATUS"=w479) -> (w472:T3)
              n211 = call-dynamic "Write SET parameters.vi"("error in (no error)"=w470, "New SET parameters"=w472, "Simulated_CCD_Camera in"=w471) -> ("error out"=w474:errorcluster, "Simulated_CCD_Camera out"=w475:refnum<class "Simulated Camera.lvclass">)  [unwired: 7 in]
              n212 = Bundle By Name(cluster=w482, "Simulated_CCD_Camera.lvclass"=w475) -> (w481:refnum<class "Channel.lvclass">)
            }
            frame "SUFFIX" {
              n213 = To Lower Case(string=w483) -> (all lower case string=w484:string)
              n214 = Bundle By Name(cluster=w487, "suffix of the image name"=w484) -> (w486:refnum<class "Channel.lvclass">)
            }
          }
          n215 = call "Write acquisition configuration.vi"("error in (no error)"=w386, "Channel in"=w387) -> ("error out"=w389:errorcluster, "Channel out"=w388:refnum<class "Channel.lvclass">)  [unwired: 8 in]
          n216 = call "Send status.vi"("error in (no error)"=w389, "Channel in"=w388) -> ("error out"=w393:errorcluster, "Channel out"=w394:refnum<class "Channel.lvclass">)  [unwired: 8 in]
          n217 = call "write state.vi"("error in (no error)"=w393, "state"="False", "Channel in"=w394) -> ("error out"=w391:errorcluster, "Channel out"=w392:refnum<class "Channel.lvclass">)  [unwired: 7 in]
        }
      }
    }
    frame Error {
    }
  }
  "error out" <- w3
  "Channel out" <- w1
